vi "Remove Diamond.vi"(8 "error in (no error)":errorcluster, 10 "Diamond to Remove":refnum<class "Diamond.lvclass">, 11 "Caves in":refnum<class "Cave.lvclass">[](array[class])) -> (0 "error out":errorcluster, 3 "Caves out":refnum<class "Cave.lvclass">[](array[class]))   [LabVIEW 2021, in "d15.lvlib" / "Cave.lvclass"]
uses:
  Cave.lvclass
  Diamond/Diamond.lvclass
  <vilib>/Analysis/geometry.llb/Point in Polygon Position.ctl
  cdcb79f0-94c4-465b-a436-5cddc884121c.vi
  324c69dd-4835-4721-a74d-aa7027ff9232.vi
  <vilib>/Analysis/geometry.llb/Point in Polygon (Array).vi
  <vilib>/Analysis/NI_AAL_Geometry.lvlib
panel:
  out "XY Graph":cluster{"X":dbl[], "Y":dbl[]}[](graph)
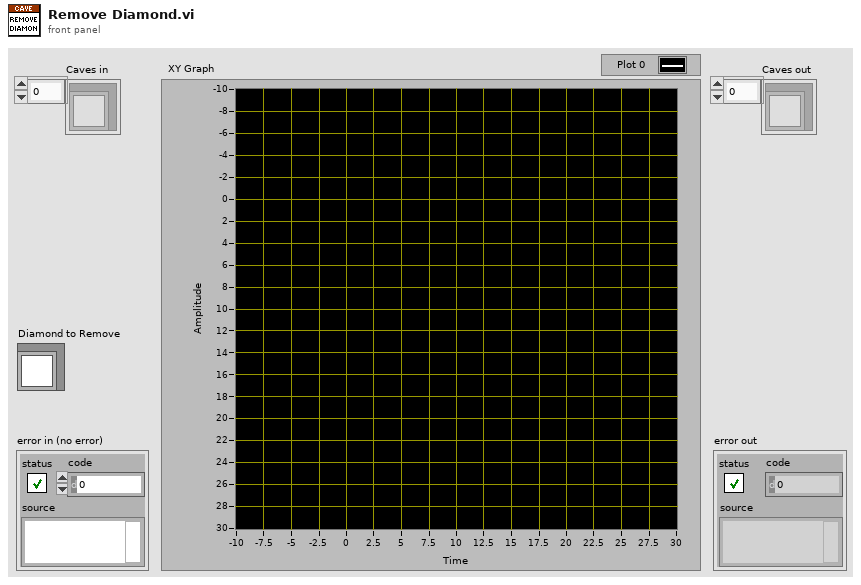
[diagram p1: front panel]
types:
  T1 = typedef "NI_AAL_Geometry.lvlib/Point in Polygon Position.ctl" = u16
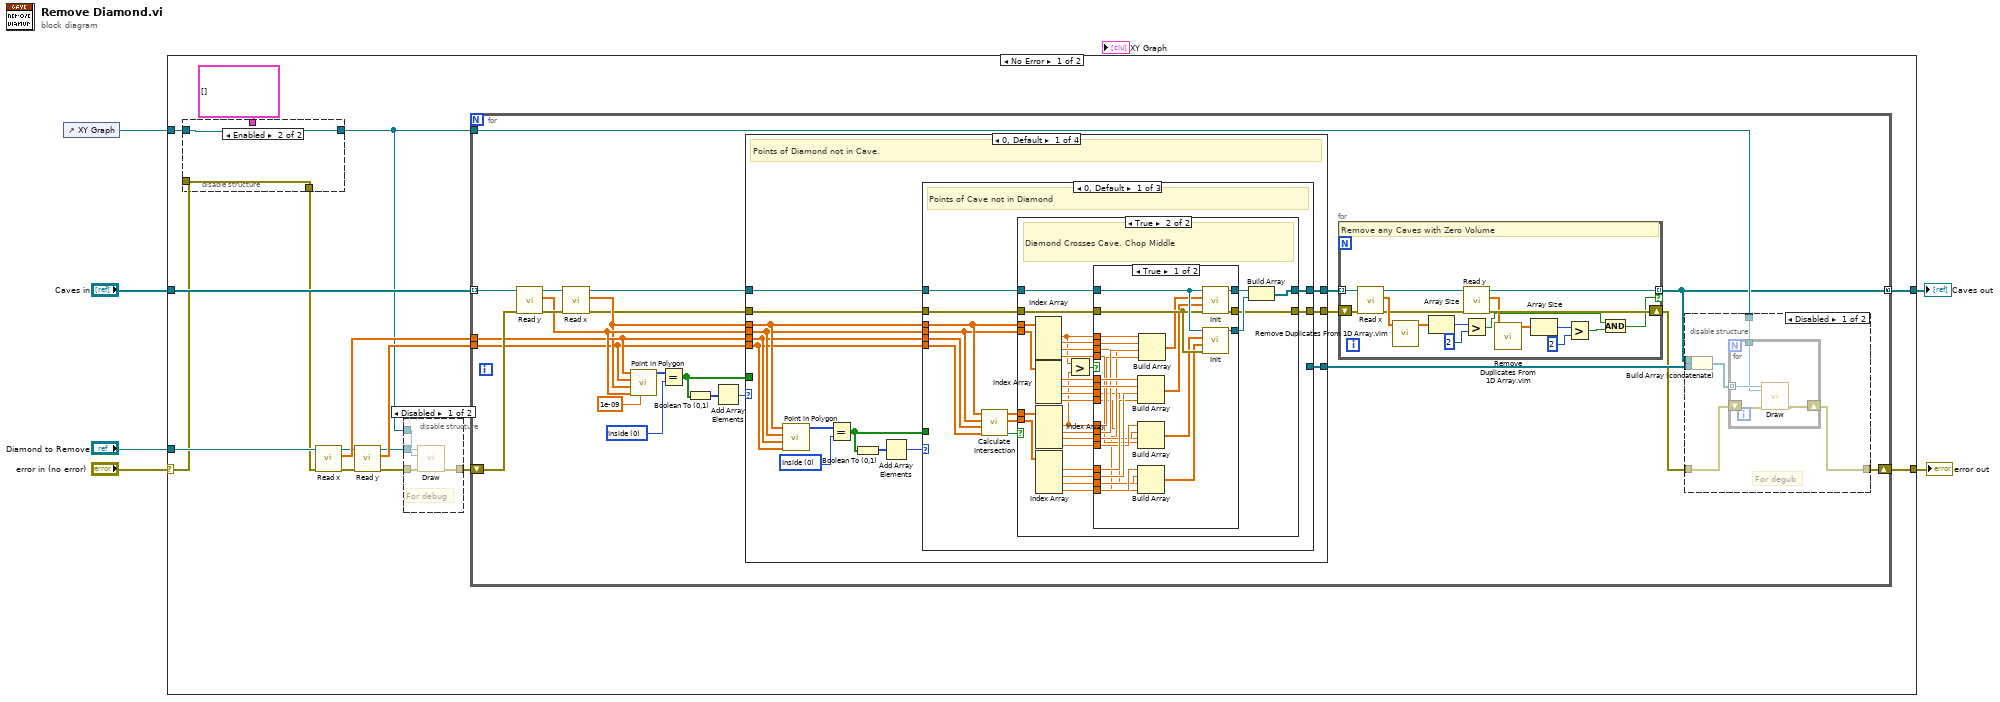
[diagram p0: block diagram]
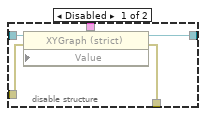
[diagram p2: hidden frame]
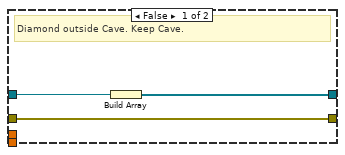
[diagram p5: hidden frame]
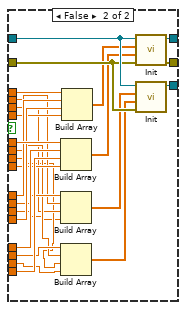
[diagram p6: hidden frame]
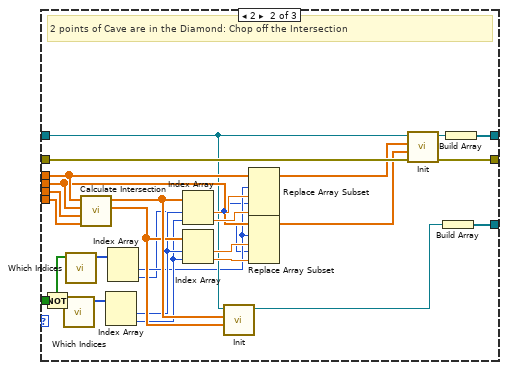
[diagram p7: hidden frame]
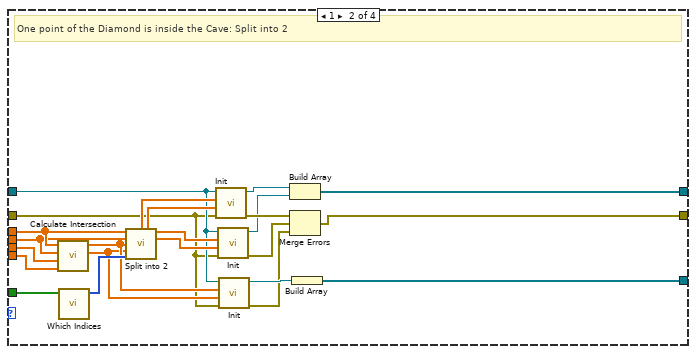
[diagram p9: hidden frame]
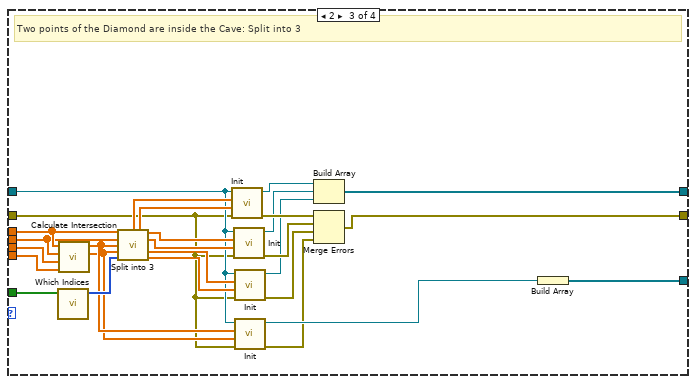
[diagram p10: hidden frame]
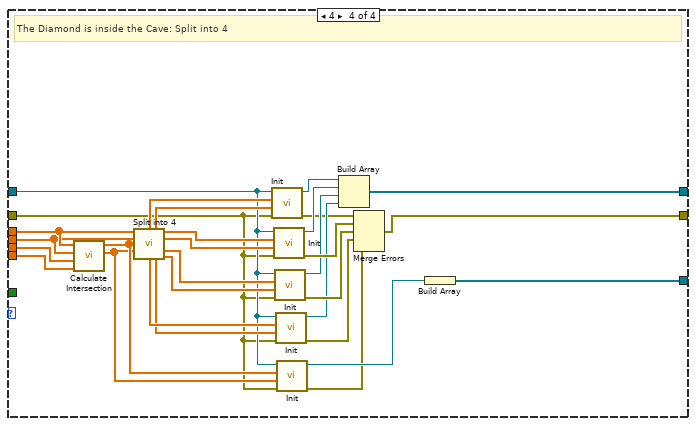
[diagram p11: hidden frame]
diagram:
  n1 = control-ref of="XY Graph"() -> (w1:refnum<vi>)
  n2 = case shown="No Error" "error in (no error)" {
    selector: "error in (no error)" -> [w10 w299]
    tunnel: [w7 w299] -> w5
    tunnel: [w11 w298] -> w2
    tunnel: "Caves in" -> [w22 w298]
    tunnel: "Diamond to Remove" -> [w20 _]
    tunnel: w1 -> [w16 _]
    frame No Error {
      n3 = disable-structure shown="Enabled" {
        disable-tunnel: w16 -> [w27 w28]
        disable-tunnel: cluster{"X":dbl[], "Y":dbl[]}[] [] ("Value") -> [w26 _]
        disable-tunnel: w10 -> [w25 w29]
        disable-tunnel: [w24 w29] -> w9
        disable-tunnel: [w23 w28] -> w8
        frame Disabled {
          n4 = property class="XYGraph (strict)"(reference=w27, error in=w25, "Value"=w26) -> (reference out=w23:refnum<vi>, error out=w24:errorcluster)
        }
        frame Enabled {
        }
      }
      n5 = call-dynamic "Read x.vi"("error in (no error)"=w9, "Diamond in"=w20) -> ("error out"=w21:errorcluster, "x"=w18:dbl[], "Diamond out"=w17:refnum<class "Diamond.lvclass">)  [unwired: 7 in]
      n6 = call-dynamic "Read y.vi"("error in (no error)"=w21, "Diamond in"=w17) -> ("error out"=w13:errorcluster, "y"=w19:dbl[], "Diamond out"=w14:refnum<class "Diamond.lvclass">)  [unwired: 7 in]
      n7 = disable-structure shown="Disabled" {
        disable-tunnel: w14 -> [w33 _]
        disable-tunnel: w13 -> [w32 w34]
        disable-tunnel: [w31 w34] -> w12
        disable-tunnel: w8 -> [w30 _]
        frame Disabled {
          # "For debug"
          n8 = call-dynamic "Draw.vi"("error in (no error)"=w32, "XY Graph"=w30, "Diamond in"=w33) -> ("error out"=w31:errorcluster)  [unwired: 7 in, 1 out]
        }
        frame Enabled {
        }
      }
      n9 = for {
        tunnel: w22 -> [w57] mode=indexing
        tunnel: [w37] -> w11 mode=concatenating
        shift-right: [w39] -> w7
        shift-left: w12 -> [w54]
        tunnel: w19 -> [w44]
        tunnel: w18 -> [w46]
        tunnel: w8 -> [w41]
        w52 = T1 0 items=["Inside", "On Boundary", "Outside"] ("x")
        n10 = call-dynamic "Read y.vi"("error in (no error)"=w54, "Diamond in"=w57) -> ("error out"=w55:errorcluster, "y"=w47:dbl[], "Diamond out"=w56:refnum<class "Cave.lvclass">)  [unwired: 7 in]
        n11 = call-dynamic "Read x.vi"("error in (no error)"=w55, "Diamond in"=w56) -> ("error out"=w43:errorcluster, "x"=w45:dbl[], "Diamond out"=w53:refnum<class "Cave.lvclass">)  [unwired: 7 in]
        n12 = call-poly <vilib>:"Point in Polygon.vi"("tolerance"=1e-09, "Polygon Y"=w47, "Polygon X"=w45, "Y"=w44, "X"=w46) -> ("Position"=w50:T1[])  [unwired: 5 in, 1 out]
        n13 = Equal?(x=w50, y=w52) -> (x = y?=w49:bool[])
        n14 = Boolean To (0,1)(Boolean=w49) -> (0, 1=w48:i16[])
        n15 = Add Array Elements(numeric array=w48) -> (sum=w51:i16)
        n16 = case shown="0, Default" w51 {
          tunnel: [w98 w236 w250 w293] -> w38
          tunnel: w53 -> [w99 w221 w247 w273]
          tunnel: w49 -> [_ w235 w255 _]
          tunnel: w45 -> [w92 w229 w254 w279]
          tunnel: w47 -> [w91 w228 w253 w278]
          tunnel: w46 -> [w90 w227 w252 w277]
          tunnel: w44 -> [w89 w226 w251 w276]
          tunnel: w43 -> [w88 w220 w242 w269]
          tunnel: [w87 w239 w244 w296] -> w36
          tunnel: [w86 w222 w245 w271] -> w40
          frame 0, Default {
            w97 = T1 0 items=["Inside", "On Boundary", "Outside"] ("x")
            # "Points of Diamond not in Cave."
            n17 = call-poly <vilib>:"Point in Polygon.vi"("Polygon Y"=w89, "Polygon X"=w90, "Y"=w91, "X"=w92) -> ("Position"=w95:T1[])  [unwired: 6 in, 1 out]
            n18 = Equal?(x=w95, y=w97) -> (x = y?=w93:bool[])
            n19 = Boolean To (0,1)(Boolean=w93) -> (0, 1=w96:i16[])
            n20 = Add Array Elements(numeric array=w96) -> (sum=w94:i16)
            n21 = case shown="0, Default" w94 {
              tunnel: w99 -> [w110 w202 _]
              tunnel: [w109 w217 _] -> w98
              tunnel: w93 -> [_ w194 _]
              tunnel: w92 -> [w101 w206 _]
              tunnel: w91 -> [w100 w205 _]
              tunnel: w90 -> [w108 w204 _]
              tunnel: w89 -> [w107 w203 _]
              tunnel: w88 -> [w103 w215 w218]
              tunnel: [w102 w214 w218] -> w87
              tunnel: [_ w198 _] -> w86
              frame 0, Default {
                # "Points of Cave not in Diamond"
                n22 = call "Calculate Intersection.vi"("Dy"=w107, "Dx"=w108, "Cy"=w100, "Cx"=w101) -> ("Found?"=w106:bool, "Y"=w104:dbl[], "X"=w105:dbl[])  [unwired: 5 in]
                n23 = case shown="True" w106 {
                  tunnel: w110 -> [w113 w138]
                  tunnel: [w112 w140] -> w109
                  tunnel: w105 -> [_ w124]
                  tunnel: w104 -> [_ w120]
                  tunnel: w103 -> [w111 w137]
                  tunnel: [w111 w114] -> w102
                  tunnel: w101 -> [_ w139]
                  tunnel: w100 -> [_ w126]
                  frame False {
                    # "Diamond outside Cave. Keep Cave."
                    n24 = Build Array(w113) -> (w112:refnum<class "Cave.lvclass">[])
                  }
                  frame True {
                    # "Diamond Crosses Cave. Chop Middle"
                    n25 = Index Array(array=w139) -> (element #1=w125:dbl, element #2=w133:dbl, element #3=w128:dbl, element #4=w127:dbl)  [unwired: 4 in]
                    n26 = Index Array(array=w126) -> (element #1=w132:dbl, element #2=w131:dbl, element #3=w130:dbl, element #4=w129:dbl)  [unwired: 4 in]
                    n27 = Index Array(array=w124) -> (element #1=w115:dbl, element #2=w123:dbl, element #3=w122:dbl, element #4=w121:dbl)  [unwired: 4 in]
                    n28 = Index Array(array=w120) -> (element #1=w119:dbl, element #2=w118:dbl, element #3=w117:dbl, element #4=w116:dbl)  [unwired: 4 in]
                    n29 = Greater?(x=w125, y=w115) -> (0:w134:bool)
                    n30 = case shown="True" w134 {
                      tunnel: w138 -> [w165 w190]
                      tunnel: w137 -> [w164 w189]
                      tunnel: [w163 w188] -> w136
                      tunnel: [w162 w187] -> w135
                      tunnel: w133 -> [w156 w172]
                      tunnel: w125 -> [w161 w182]
                      tunnel: w132 -> [w159 w181]
                      tunnel: w131 -> [w155 w171]
                      tunnel: w130 -> [w143 w169]
                      tunnel: w129 -> [w142 w175]
                      tunnel: w128 -> [w145 w170]
                      tunnel: w127 -> [w144 w176]
                      tunnel: w115 -> [w151 w180]
                      tunnel: w123 -> [w153 w174]
                      tunnel: w122 -> [w146 w168]
                      tunnel: w121 -> [w149 w178]
                      tunnel: w119 -> [w150 w179]
                      tunnel: w118 -> [w152 w173]
                      tunnel: w117 -> [w147 w167]
                      tunnel: w116 -> [w148 w177]
                      tunnel: [w141 w166] -> w114
                      frame True {
                        n31 = Build Array(w159, w155, w152, w150) -> (w154:dbl[])
                        n32 = Build Array(w149, w146, w145, w144) -> (w158:dbl[])
                        n33 = Build Array(w148, w147, w143, w142) -> (w157:dbl[])
                        n34 = Build Array(w161, w156, w153, w151) -> (w160:dbl[])
                        n35 = call-dynamic "Init.vi"("error in (no error)"=w164, "y"=w154, "x"=w160, "Diamond in"=w165) -> ("error out"=w141:errorcluster, "Diamond out"=w163:refnum<class "Cave.lvclass">)  [unwired: 6 in]
                        n36 = call-dynamic "Init.vi"("error in (no error)"=w164, "y"=w157, "x"=w158, "Diamond in"=w165) -> ("Diamond out"=w162:refnum<class "Cave.lvclass">)  [unwired: 6 in, 1 out]
                      }
                      frame False {
                        n37 = Build Array(w181, w179, w177, w175) -> (w183:dbl[])
                        n38 = Build Array(w174, w172, w170, w168) -> (w185:dbl[])
                        n39 = Build Array(w173, w171, w169, w167) -> (w184:dbl[])
                        n40 = Build Array(w182, w180, w178, w176) -> (w186:dbl[])
                        n41 = call-dynamic "Init.vi"("error in (no error)"=w189, "y"=w183, "x"=w186, "Diamond in"=w190) -> ("error out"=w166:errorcluster, "Diamond out"=w188:refnum<class "Cave.lvclass">)  [unwired: 6 in]
                        n42 = call-dynamic "Init.vi"("error in (no error)"=w189, "y"=w184, "x"=w185, "Diamond in"=w190) -> ("Diamond out"=w187:refnum<class "Cave.lvclass">)  [unwired: 6 in, 1 out]
                      }
                    }
                    n43 = Build Array(w136, w135) -> (w140:refnum<class "Cave.lvclass">[])
                  }
                }
              }
              frame 2 {
                # "2 points of Cave are in the Diamond: Chop off the Intersection"
                n44 = Not(x=w194) -> (.not. x?=w197:bool[])
                n45 = call "Which Indices.vi"("In"=w197) -> ("X"=w207:u8[])  [unwired: 10 in]
                n46 = call "Which Indices.vi"("In"=w194) -> ("X"=w193:u8[])  [unwired: 10 in]
                n47 = call "Calculate Intersection.vi"("Dy"=w203, "Dx"=w204, "Cy"=w205, "Cx"=w206) -> ("Y"=w200:dbl[], "X"=w201:dbl[])  [unwired: 5 in, 1 out]
                n48 = Index Array(array=w207) -> (element #1=w196:u8, element #2=w195:u8)  [unwired: 2 in]
                n49 = Index Array(array=w193) -> (element #1=w192:u8, element #2=w191:u8)  [unwired: 2 in]
                n50 = Index Array(array=w201, index #1=w196, index #2=w195) -> (element #1=w213:dbl, element #2=w210:dbl)
                n51 = Index Array(array=w200, index #1=w196, index #2=w195) -> (element #1=w212:dbl, element #2=w211:dbl)
                n52 = call-dynamic "Init.vi"("y"=w200, "x"=w201, "Diamond in"=w202) -> ("Diamond out"=w199:refnum<class "Cave.lvclass">)  [unwired: 7 in, 1 out]
                n53 = Replace Array Subset(array=w206, new element #1=w213, index #1=w192, new element #2=w210, index #2=w191) -> (w209:dbl[])
                n54 = Replace Array Subset(array=w205, new element #1=w212, index #1=w192, new element #2=w211, index #2=w191) -> (w208:dbl[])
                n55 = call-dynamic "Init.vi"("error in (no error)"=w215, "y"=w208, "x"=w209, "Diamond in"=w202) -> ("error out"=w214:errorcluster, "Diamond out"=w216:refnum<class "Cave.lvclass">)  [unwired: 6 in]
                n56 = Build Array(w199) -> (w198:refnum<class "Cave.lvclass">[])
                n57 = Build Array(w216) -> (w217:refnum<class "Cave.lvclass">[])
              }
              frame 4 {
                # "Cave is in Diamond, Delete Cave"
              }
            }
          }
          frame 1 {
            # "One point of the Diamond is inside the Cave: Split into 2"
            n58 = call "Calculate Intersection.vi"("Dy"=w226, "Dx"=w227, "Cy"=w228, "Cx"=w229) -> ("Y"=w224:dbl[], "X"=w225:dbl[])  [unwired: 5 in, 1 out]
            n59 = call "Which Indices.vi"("In"=w235) -> ("X"=w234:u8[])  [unwired: 10 in]
            n60 = call "Split into 2.vi"("Cx"=w229, "Cy"=w228, "Ix"=w225, "Iy"=w224, "X"=w234) -> ("C1x"=w233:dbl[], "C1y"=w232:dbl[], "C2x"=w231:dbl[], "C2y"=w230:dbl[])  [unwired: 7 in]
            n61 = call-dynamic "Init.vi"("error in (no error)"=w220, "y"=w232, "x"=w233, "Diamond in"=w221) -> ("error out"=w241:errorcluster, "Diamond out"=w238:refnum<class "Cave.lvclass">)  [unwired: 6 in]
            n62 = call-dynamic "Init.vi"("error in (no error)"=w220, "y"=w230, "x"=w231, "Diamond in"=w221) -> ("error out"=w240:errorcluster, "Diamond out"=w237:refnum<class "Cave.lvclass">)  [unwired: 6 in]
            n63 = call-dynamic "Init.vi"("error in (no error)"=w220, "y"=w224, "x"=w225, "Diamond in"=w221) -> ("error out"=w219:errorcluster, "Diamond out"=w223:refnum<class "Cave.lvclass">)  [unwired: 6 in]
            n64 = Build Array(w238, w237) -> (w236:refnum<class "Cave.lvclass">[])
            n65 = Merge Errors(w241, w240, w219) -> (w239:errorcluster)
            n66 = Build Array(w223) -> (w222:refnum<class "Cave.lvclass">[])
          }
          frame 2 {
            # "Two points of the Diamond are inside the Cave: Split into 3"
            n67 = call "Which Indices.vi"("In"=w255) -> ("X"=w264:u8[])  [unwired: 10 in]
            n68 = call "Calculate Intersection.vi"("Dy"=w251, "Dx"=w252, "Cy"=w253, "Cx"=w254) -> ("Y"=w248:dbl[], "X"=w249:dbl[])  [unwired: 5 in, 1 out]
            n69 = call "Split into 3.vi"("Cx"=w254, "Cy"=w253, "Ix"=w249, "Iy"=w248, "X"=w264) -> ("C1x"=w260:dbl[], "C1y"=w259:dbl[], "C2x"=w258:dbl[], "C2y"=w257:dbl[], "C3x"=w261:dbl[], "C3y"=w256:dbl[])  [unwired: 5 in]
            n70 = call-dynamic "Init.vi"("error in (no error)"=w242, "y"=w259, "x"=w260, "Diamond in"=w247) -> ("error out"=w268:errorcluster, "Diamond out"=w266:refnum<class "Cave.lvclass">)  [unwired: 6 in]
            n71 = call-dynamic "Init.vi"("error in (no error)"=w242, "y"=w257, "x"=w258, "Diamond in"=w247) -> ("error out"=w267:errorcluster, "Diamond out"=w265:refnum<class "Cave.lvclass">)  [unwired: 6 in]
            n72 = call-dynamic "Init.vi"("error in (no error)"=w242, "y"=w256, "x"=w261, "Diamond in"=w247) -> ("error out"=w262:errorcluster, "Diamond out"=w263:refnum<class "Cave.lvclass">)  [unwired: 6 in]
            n73 = call-dynamic "Init.vi"("error in (no error)"=w242, "y"=w248, "x"=w249, "Diamond in"=w247) -> ("error out"=w243:errorcluster, "Diamond out"=w246:refnum<class "Cave.lvclass">)  [unwired: 6 in]
            n74 = Build Array(w266, w265, w263) -> (w250:refnum<class "Cave.lvclass">[])
            n75 = Merge Errors(w268, w267, w262, w243) -> (w244:errorcluster)
            n76 = Build Array(w246) -> (w245:refnum<class "Cave.lvclass">[])
          }
          frame 4 {
            # "The Diamond is inside the Cave: Split into 4"
            n77 = call "Calculate Intersection.vi"("Dy"=w276, "Dx"=w277, "Cy"=w278, "Cx"=w279) -> ("Y"=w274:dbl[], "X"=w275:dbl[])  [unwired: 5 in, 1 out]
            n78 = call "Split into 4.vi"("Cx"=w279, "Cy"=w278, "Ix"=w275, "Iy"=w274) -> ("C1x"=w289:dbl[], "C1y"=w288:dbl[], "C2x"=w287:dbl[], "C2y"=w292:dbl[], "C3x"=w286:dbl[], "C4x"=w282:dbl[], "C4y"=w281:dbl[], "C3y"=w285:dbl[])  [unwired: 4 in]
            n79 = call-dynamic "Init.vi"("error in (no error)"=w269, "y"=w288, "x"=w289, "Diamond in"=w273) -> ("error out"=w283:errorcluster, "Diamond out"=w295:refnum<class "Cave.lvclass">)  [unwired: 6 in]
            n80 = call-dynamic "Init.vi"("error in (no error)"=w269, "y"=w292, "x"=w287, "Diamond in"=w273) -> ("error out"=w297:errorcluster, "Diamond out"=w294:refnum<class "Cave.lvclass">)  [unwired: 6 in]
            n81 = call-dynamic "Init.vi"("error in (no error)"=w269, "y"=w285, "x"=w286, "Diamond in"=w273) -> ("error out"=w290:errorcluster, "Diamond out"=w291:refnum<class "Cave.lvclass">)  [unwired: 6 in]
            n82 = call-dynamic "Init.vi"("error in (no error)"=w269, "y"=w281, "x"=w282, "Diamond in"=w273) -> ("error out"=w280:errorcluster, "Diamond out"=w284:refnum<class "Cave.lvclass">)  [unwired: 6 in]
            n83 = call-dynamic "Init.vi"("error in (no error)"=w269, "y"=w274, "x"=w275, "Diamond in"=w273) -> ("error out"=w270:errorcluster, "Diamond out"=w272:refnum<class "Cave.lvclass">)  [unwired: 6 in]
            n84 = Build Array(w295, w294, w291, w284) -> (w293:refnum<class "Cave.lvclass">[])
            n85 = Merge Errors(w283, w297, w290, w280, w270) -> (w296:errorcluster)
            n86 = Build Array(w272) -> (w271:refnum<class "Cave.lvclass">[])
          }
        }
        n87 = for {
          tunnel: w38 -> [w74] mode=indexing
          tunnel: [w67] -> w37 mode=indexing if=w58
          shift-right: [w65] -> w35
          shift-left: w36 -> [w72]
          # "Remove any Caves with Zero Volume"
          n88 = call-dynamic "Read x.vi"("error in (no error)"=w72, "Diamond in"=w74) -> ("error out"=w66:errorcluster, "x"=w71:dbl[], "Diamond out"=w73:refnum<class "Cave.lvclass">)  [unwired: 7 in]
          n89 = call "Remove Duplicates From 1D Array.vim"("array"=w71) -> ("array with duplicates removed"=w70:dbl[])  [unwired: 10 in]
          n90 = Array Size(array=w70) -> (size(s)=w69:i32)
          n91 = call-dynamic "Read y.vi"("error in (no error)"=w66, "Diamond in"=w73) -> ("error out"=w65:errorcluster, "y"=w63:dbl[], "Diamond out"=w67:refnum<class "Cave.lvclass">)  [unwired: 7 in]
          n92 = Greater?(x=w69, y=2) -> (0:w59:bool)
          n93 = call "Remove Duplicates From 1D Array.vim"("array"=w63) -> ("array with duplicates removed"=w62:dbl[])  [unwired: 10 in]
          n94 = Array Size(array=w62) -> (size(s)=w61:i32)
          n95 = Greater?(x=w61, y=2) -> (0:w60:bool)
          n96 = And(x=w59, y=w60) -> (x .and. y?=w58:bool)
        }
        n97 = disable-structure shown="Disabled" {
          disable-tunnel: w41 -> [w80 _]
          disable-tunnel: [w79 w85] -> w39
          disable-tunnel: w37 -> [w78 _]
          disable-tunnel: w40 -> [w77 _]
          disable-tunnel: w35 -> [w75 w85]
          frame Disabled {
            # "For degub"
            n98 = Build Array (concatenate)(w78, w77) -> (w76:refnum<class "Cave.lvclass">[])
            n99 = for {
              tunnel: w76 -> [w84] mode=indexing
              tunnel: w80 -> [w83]
              shift-right: [w81] -> w79
              shift-left: w75 -> [w82]
              n100 = call-dynamic "Draw.vi"("error in (no error)"=w82, "XY Graph"=w83, "Diamond in"=w84) -> ("error out"=w81:errorcluster)  [unwired: 7 in, 1 out]
            }
          }
          frame Enabled {
          }
        }
      }
    }
    frame Error {
    }
  }
  "error out" <- w5
  "Caves out" <- w2
